vi "Copyright.vi"() -> (3 "String":string)   [LabVIEW 2025]
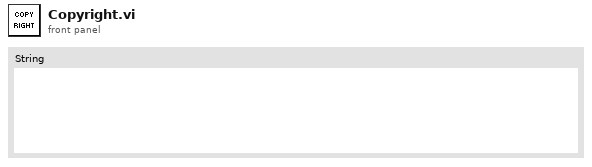
[diagram p1: front panel]
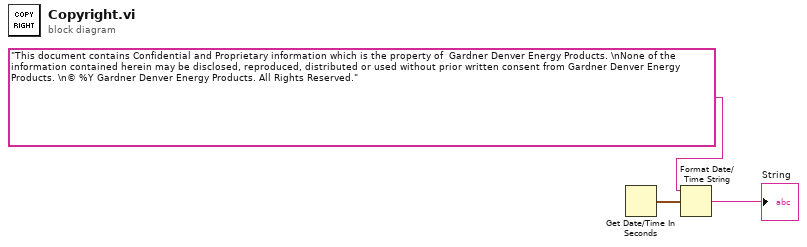
[diagram p0: block diagram]
diagram:
  n1 = Get Date/Time In Seconds() -> (seconds since 1Jan1904=w2:timestamp)
  n2 = Format Date/Time String(time format string (%c)="This document contains Confidential and Proprietary information which is the property of  Gardner Denver Energy Products. \nNone of the information contained herein may be disclosed, reproduced, distributed or used without prior written consent from Gardner Denver Energy Products. \n© %Y Gardner Denver Energy Products. All Rights Reserved." ("format string"), seconds (now)=w2) -> (date/time string=→"String":string)  [unwired: 1 in]
